vi "录音.vi"() -> ()   [LabVIEW 2018]
uses:
  <vilib>/sound2/lvsound2.llb/Sound Data Format.ctl
  <vilib>/sound2/lvsound2.llb/Sampling Mode.ctl
  <vilib>/sound2/lvsound2.llb/Sound File Write Open.vi
  <vilib>/sound2/lvsound2.llb/Sound Input Read (DBL).vi
  <vilib>/sound2/lvsound2.llb/Sound File Write (DBL).vi
panel:
  in  "停止":bool
  out "波形图":waveform(dbl)[](graph)
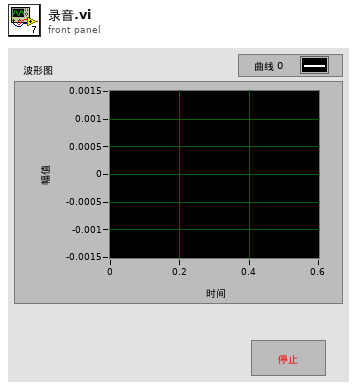
[diagram p1: front panel]
types:
  T1 = typedef "Sampling Mode.ctl" = i32
  T2 = typedef "Sound Data Format.ctl" = cluster{"sample rate (S/s)":dbl, "number of channels":i32, "bits per sample":i32}
  T3 = typedef "Sound File Refnum.ctl" = refnum<file>
  T4 = typedef "Sound Input Task ID.ctl" = u32
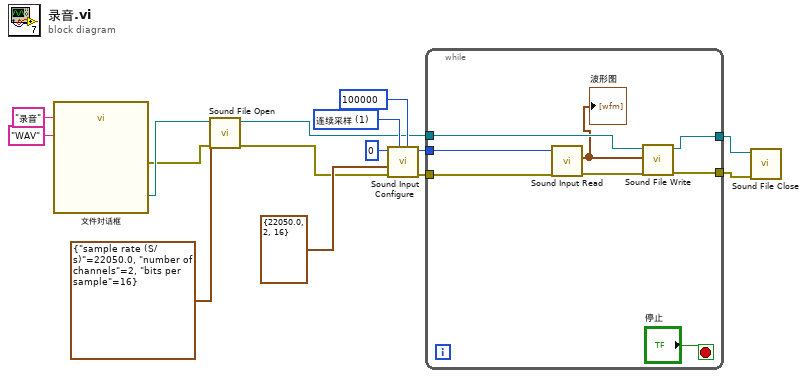
[diagram p0: block diagram]
diagram:
  w8 = T1 1 items=["有限采样", "连续采样"] ("sample mode")
  n1 = call "文件对话框"("default name"="录音", "pattern (all files)"="WAV") -> ("selected path"=w13:path, "error out"=w9:errorcluster)  [unwired: 10 in, 2 out]
  n2 = call-poly <vilib>:"Sound File Open.vi"("error in (no error)"=w9, "sound format"=T2 {"sample rate (S/s)"=22050.0, "number of channels"=2, "bits per sample"=16}, "path"=w13) -> ("error out"=w10:errorcluster, "sound file refnum"=w3:T3)  [unwired: 7 in]
  n3 = call <vilib>:"Sound Input Configure.vi"("number of samples/ch"=100000, "sample mode"=w8, "error in (no error)"=w10, "sound format"=T2 {"sample rate (S/s)"=22050.0, "number of channels"=2, "bits per sample"=16}, "device ID"=u32 0) -> ("error out"=w4:errorcluster, "task ID"=w5:T4)  [unwired: 5 in]
  n4 = while {
    tunnel: w5 -> [w23]
    tunnel: w4 -> [w22]
    tunnel: w3 -> [w21]
    tunnel: [w19] -> w1
    tunnel: [w18] -> w2
    stop <- "停止" stop-if-true
    n5 = call-poly <vilib>:"Sound Input Read.vi"("error in (no error)"=w22, "task ID"=w23) -> ("error out"=w20:errorcluster, "data"=w17:waveform(dbl)[])  [unwired: 7 in, 1 out]
    "波形图" <- w17
    n6 = call-poly <vilib>:"Sound File Write.vi"("error in (no error)"=w20, "data"=w17, "sound file refnum"=w21) -> ("error out"=w18:errorcluster, "sound file refnum out"=w19:T3)  [unwired: 7 in]
  }
  n7 = call <vilib>:"Sound File Close.vi"("error in (no error)"=w2, "sound file refnum"=w1) -> ()  [unwired: 9 in, 1 out]
